vi "XML double.vi"(8 "tag":string, 11 "String":string) -> (3 "int":dbl)   [LabVIEW 2013]
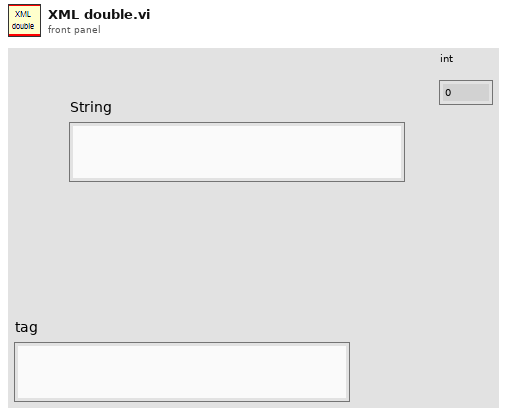
[diagram p1: front panel]
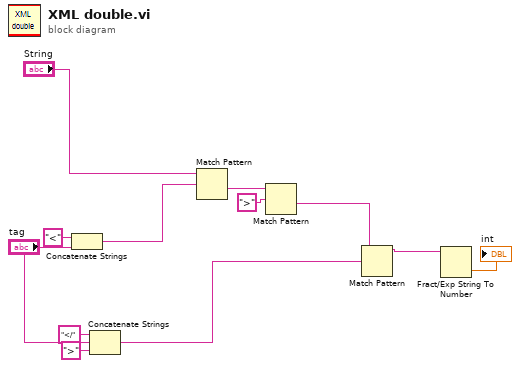
[diagram p0: block diagram]
diagram:
  n1 = Concatenate Strings("<" ("string"), "tag") -> (w4:string)
  n2 = Concatenate Strings("</" ("string"), "tag", ">" ("string")) -> (w3:string)
  n3 = Match Pattern(string="String", regular expression=w4) -> (after substring=w11:string)  [unwired: 1 in, 3 out]
  n4 = Match Pattern(string=w11, regular expression=">") -> (after substring=w9:string)  [unwired: 1 in, 3 out]
  n5 = Match Pattern(string=w9, regular expression=w3) -> (before substring=w2:string)  [unwired: 1 in, 3 out]
  n6 = Fract/Exp String To Number(string=w2) -> (number=→"int":dbl)  [unwired: 3 in, 1 out]
